vi "Get Unbundler Output Terminal Names.vi"(8 "error in (no error)":errorcluster, 11 "Unbundler in":refnum<vi>) -> (0 "error out":errorcluster, 2 "Terminal names":string[](array[string]), 3 "Unbundler out":refnum<vi>)   [LabVIEW 2019, in "gRPC Template Creation Utility.lvlib"]
uses:
  gRPC Template Creation Utility.lvlib
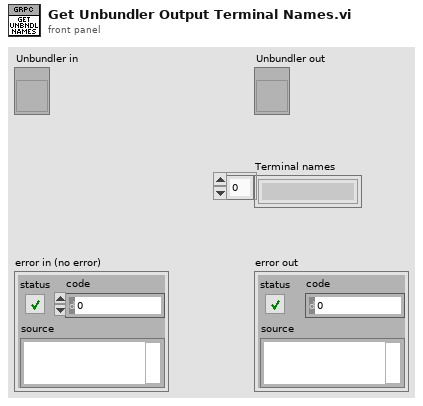
[diagram p1: front panel]
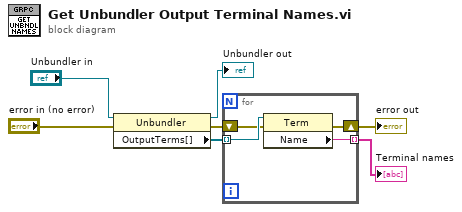
[diagram p0: block diagram]
diagram:
  n1 = property class="Unbundler"(reference="Unbundler in", error in="error in (no error)") -> (reference out=→"Unbundler out":refnum<vi>, error out=w6:errorcluster, "OutputTerms[]"=w4:refnum<vi>[])
  n2 = for {
    tunnel: w4 -> [w11] mode=indexing
    tunnel: [w10] -> w7 mode=indexing
    shift-right: [w8] -> w2
    shift-left: w6 -> [w9]
    n3 = property class="Term"(reference=w11, error in=w9) -> (error out=w8:errorcluster, "Name"=w10:string)  [unwired: 1 out]
  }
  "Terminal names" <- w7
  "error out" <- w2
